vi "3-3.vi"(0 "偏移量(0)":i32, 1 "长度（剩余）":i32, 2 "字符串":string, 3 "偏移量(0) 2":i32, 4 "长度（剩余） 2":i32, 5 "偏移量(0) 3":i32, 6 "长度（剩余） 3":i32) -> (7 "输出 1":dbl, 8 "子字符串":string, 9 "子字符串 2":string)   [LabVIEW 2017]
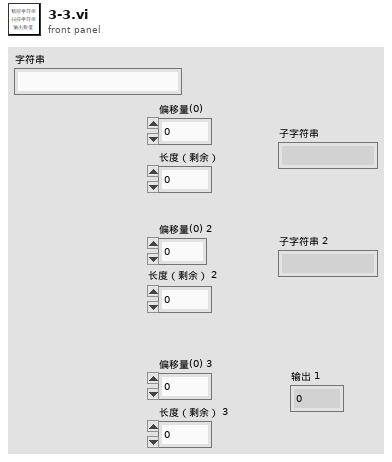
[diagram p1: front panel]
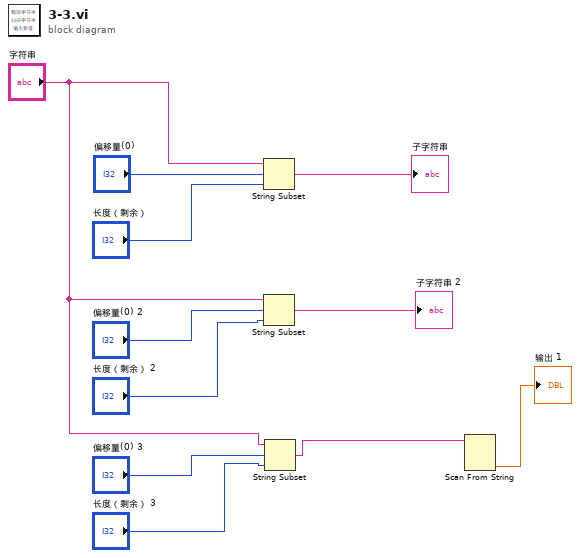
[diagram p0: block diagram]
diagram:
  n1 = String Subset(string="字符串", offset (0)="偏移量(0)", length (rest)="长度（剩余）") -> (substring=→"子字符串":string)
  n2 = String Subset(string="字符串", offset (0)="偏移量(0) 2", length (rest)="长度（剩余） 2") -> (substring=→"子字符串 2":string)
  n3 = String Subset(string="字符串", offset (0)="偏移量(0) 3", length (rest)="长度（剩余） 3") -> (substring=w2:string)
  n4 = Scan From String(input string=w2) -> (output 1=→"输出 1":dbl)  [unwired: 4 in, 3 out]
